vi "broadcastReg-TestCore.vi"(7 "status":string="status@source >> api@target -><register>\nstatus@source >> api2@target -><register>", 9 "Target":string="target", 10 "Source":string="source", 11 "Status":string="status") -> (3 "Response Message Info":T1[](array[typedef]))   [LabVIEW 2017, in "testcase-Broadcast Registry.lvclass"]
uses:
  testcase-Broadcast Registry.lvclass
  src/user.lib/_NEVSTOP/Communicable State Machine(CSM)/_Support/BroadcastRegistry/BroadcastRegistry-Value.ctl
  src/user.lib/_NEVSTOP/Communicable State Machine(CSM)/AdvanceAPI/CSM - Broadcast Message Type.ctl
  src/user.lib/_NEVSTOP/Communicable State Machine(CSM)/Communicable State Machine.lvlib
  src/user.lib/_NEVSTOP/Communicable State Machine(CSM)/_Shared/CSM Shared.lvlib
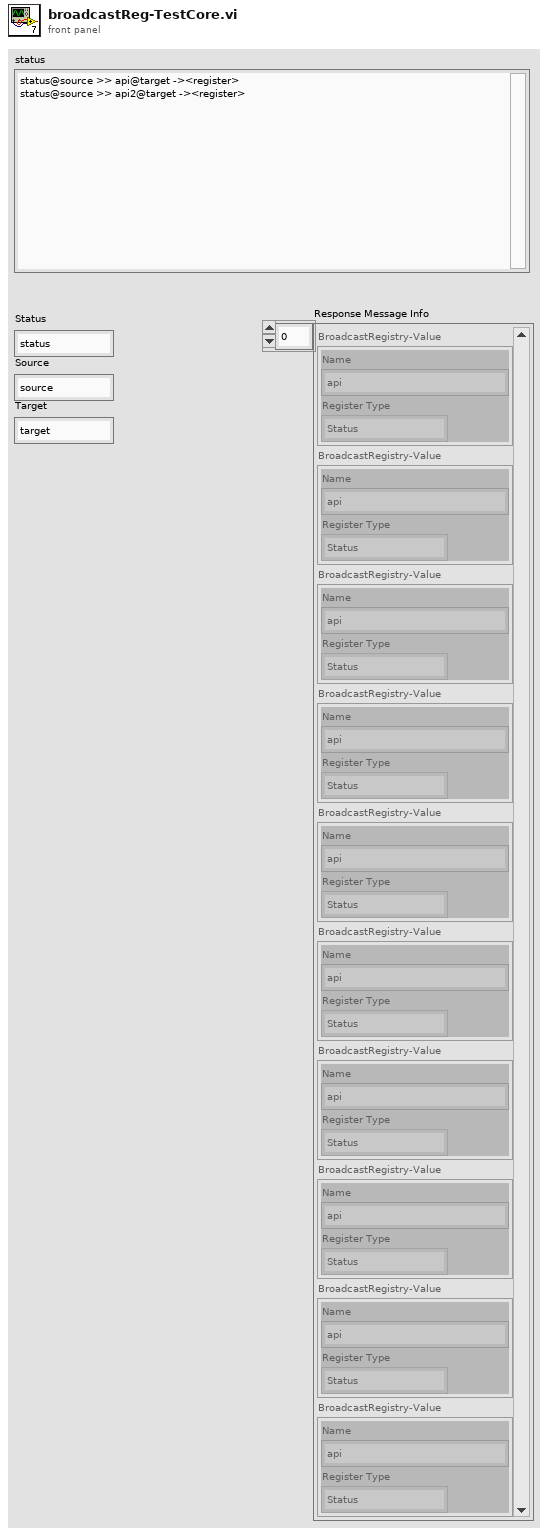
[diagram p1: front panel]
types:
  T1 = typedef "Communicable State Machine.lvlib/BroadcastRegistry-Value.ctl" = cluster{"Name":string, "Register Type":T2}
  T2 = typedef "Communicable State Machine.lvlib/CSM - Broadcast Message Type.ctl" = enum16{"<Null>", "Status", "Interrupt"}
  T3 = typedef "Communicable State Machine.lvlib/BroadcastRegistry.ctl" = cluster{"RegistryTable":variant}
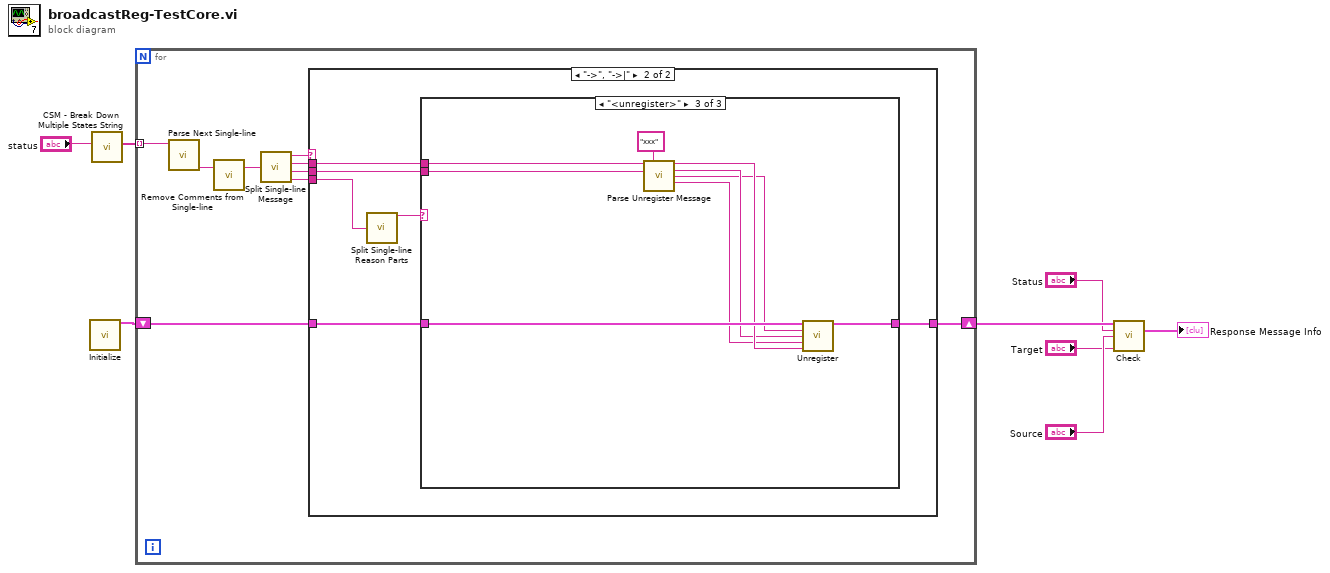
[diagram p0: block diagram]
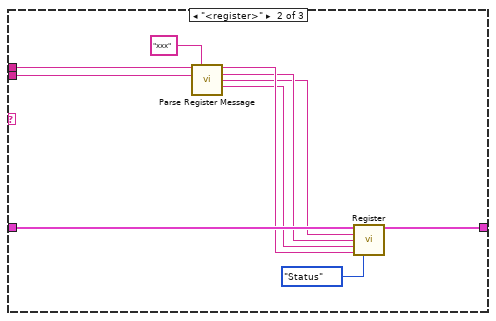
[diagram p4: hidden frame]
diagram:
  n1 = call "Initialize.vi"() -> ("BroadcastRegistry Out"=w6:T3)  [unwired: 15 in]
  n2 = call "CSM - Break Down Multiple States String.vi"("States"="status") -> ("Multiple States"=w7:string[])  [unwired: 10 in]
  n3 = for {
    tunnel: w7 -> [w15] mode=indexing
    shift-right: [w9] -> w5
    shift-left: w6 -> [w10]
    n4 = call "Parse Next Single-line.vi"("States Queue"=w15) -> ("Next Single-line State"=w16:string)  [unwired: 9 in, 1 out]
    n5 = call "Remove Comments from Single-line.vi"("single-line text"=w16) -> ("single-line text without comments"=w17:string)  [unwired: 2 in]
    n6 = call "Split Single-line Message.vi"("single-line text"=w17) -> ("operator"=w14:string, "state"=w13:string, "args"=w12:string, "source/target"=w11:string)  [unwired: 6 in]
    n7 = case shown="\"->\", \"->|\"" w14 {
      tunnel: w13 -> [_ w24]
      tunnel: w12 -> [_ w23]
      tunnel: w11 -> [_ w20]
      tunnel: w10 -> [w18 w22]
      tunnel: [w18 w21] -> w9
      frame "False", Default {
      }
      frame "->", "->|" {
        n8 = call "Split Single-line Reason Parts.vi"("Single-line -& Reason"=w20) -> ("CSM Name"=w19:string)  [unwired: 12 in, 2 out]
        n9 = case shown="\"<unregister>\"" w19 {
          tunnel: w24 -> [_ w32 w41]
          tunnel: w23 -> [_ w31 w40]
          tunnel: w22 -> [w25 w35 w44]
          tunnel: [w25 w34 w43] -> w21
          frame "False", Default {
          }
          frame "<register>" {
            n10 = call "Parse Register Message.vi"("State"=w32, "Module Name"="xxx", "Args"=w31) -> ("Target"=w30:string, "Source"=w29:string, "Status"=w28:string, "Api"=w27:string)  [unwired: 8 in, 1 out]
            n11 = call "Register.vi"("BroadcastRegistry In"=w35, "Broadcast"=w28, "SourceCSM"=w29, "Name"=w27, "TargetCSM"=w30, "Register Type"=CSM_-_Broadcast_Message_Type."Status" ("Priority")) -> ("BroadcastRegistry Out"=w34:T3)  [unwired: 9 in]
          }
          frame "<unregister>" {
            n12 = call "Parse Unregister Message.vi"("State"=w41, "Module Name"="xxx", "Args"=w40) -> ("Target"=w39:string, "Source"=w38:string, "Status"=w37:string, "Api"=w36:string)  [unwired: 8 in, 1 out]
            n13 = call "Unregister.vi"("BroadcastRegistry In"=w44, "Broadcast"=w37, "SourceCSM"=w38, "API"=w36, "TargetCSM"=w39) -> ("BroadcastRegistry Out"=w43:T3)  [unwired: 10 in]
          }
        }
      }
    }
  }
  n14 = call "Check.vi"("BroadcastRegistry In"=w5, "Broadcast"="Status", "SourceCSM"="Source", "TargetCSM"="Target") -> ("Response Message Info"=→"Response Message Info":T1[])  [unwired: 10 in, 1 out]
